vi "StateMachineDAQ.vi"() -> ()   [LabVIEW 2014]
doc: "Use this template to build a user interface event handler design pattern. Use this pattern for dialog boxes and other user interfaces. You also can create and execute user-defined events that the VI can handle the same way as user interface events."
uses:
  subVIs/StateMachineDAQState.ctl
  <vilib>/Utility/error.llb/DialogType.ctl
  <vilib>/DAQmx/create/channels.llb/DAQmx Create Channel (AI-Voltage-Basic).vi
  <vilib>/DAQmx/configure/timing.llb/DAQmx Timing (Sample Clock).vi
  <vilib>/DAQmx/read.llb/DAQmx Read (Analog Wfm 1Chan NSamp).vi
  <resource>/objmgr/daqmx.rc
panel:
  in  "File Path":path
  in  "Acquire Data":bool
  in  "Log Data":bool
  in  "File Comment":string
  in  "DAQ Parameters":T1={"physical channels"="", "maximum value"=5.0, "minimum value"=-5.0, "rate"=1000.0, "read period"=0.5} {"read period" format="%0.2f"; "rate" format="%0.2f"; "minimum value" format="%0.2f"; "maximum value" format="%0.2f"}
  out "Waveform Chart":waveform(dbl)(graph)
  in  "quit":bool
  # "V"
  # "V"
  # "Hz"
  # "s"
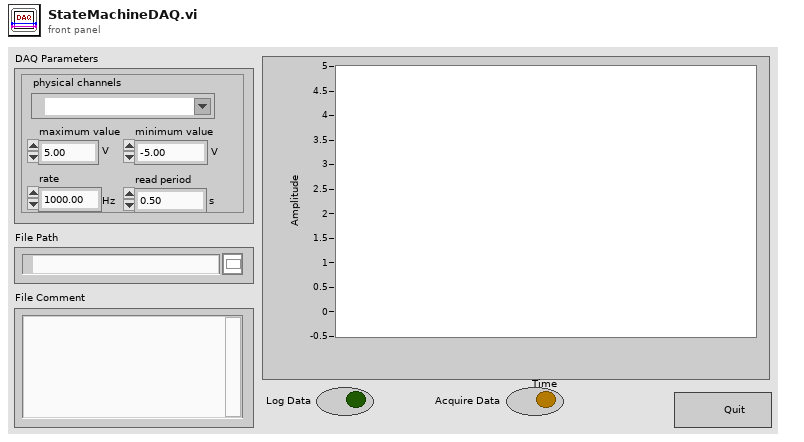
[diagram p1: front panel]
types:
  T1 = cluster{"physical channels":tag, "maximum value":dbl, "minimum value":dbl, "rate":dbl, "read period":dbl}
  T2 = typedef "StateMachineDAQState.ctl" = enum16{"Init", "Idle", "CheckError", "Finalize", "ConfigDAQ", "StartDAQ", "AcquireAndLog", "StopDAQ", "ClearDAQ", "OpenFile", "CloseFile", "Process 1"}
  T3 = typedef "DialogType.ctl" = u16
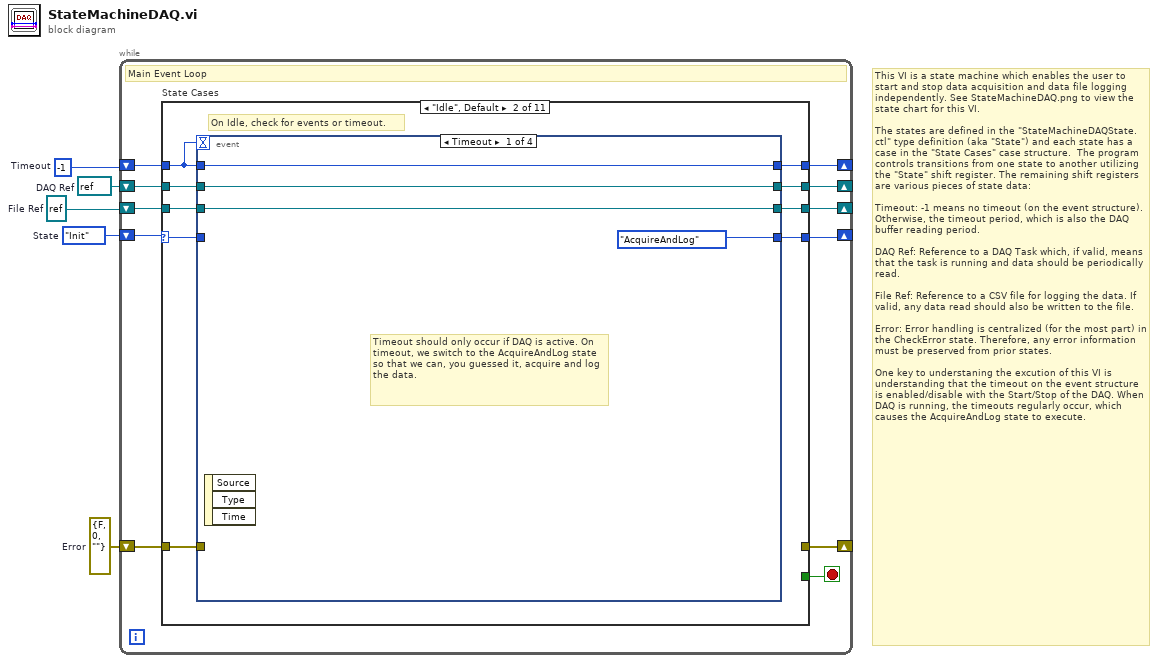
[diagram p0: block diagram]
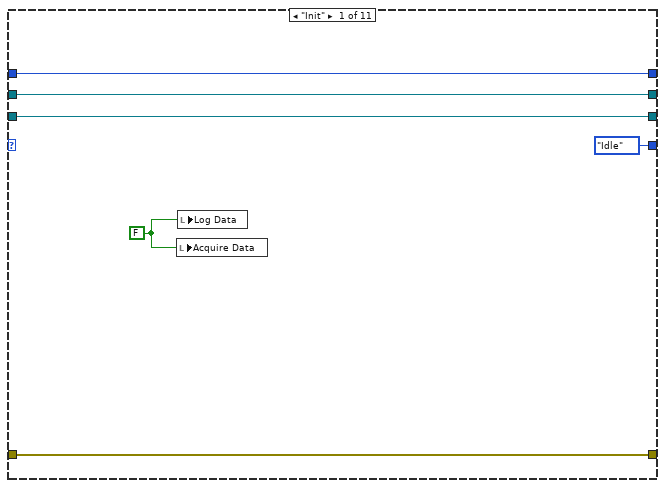
[diagram p2: hidden frame]
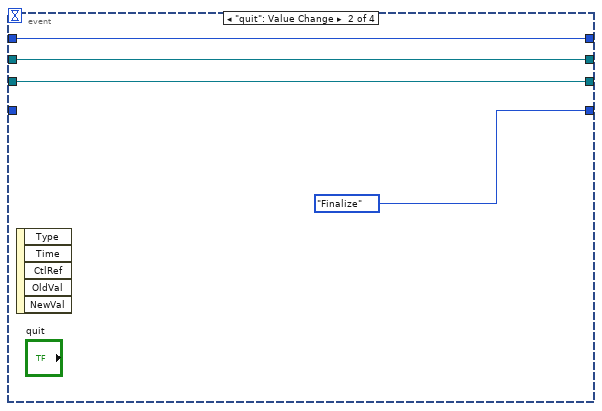
[diagram p3: hidden frame]
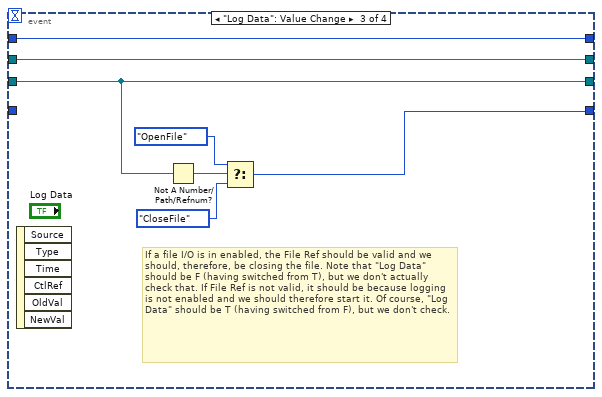
[diagram p4: hidden frame]
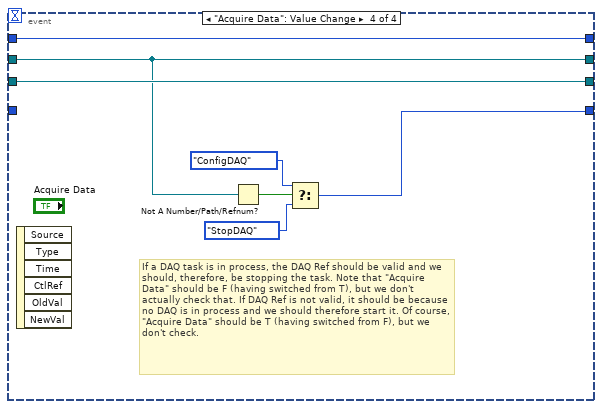
[diagram p5: hidden frame]
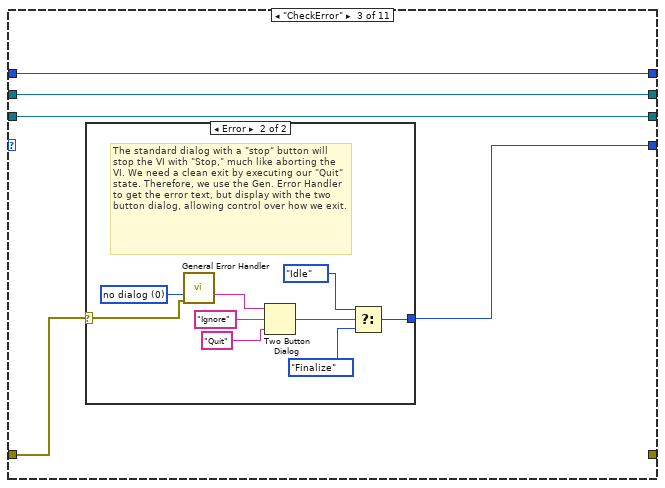
[diagram p6: hidden frame]
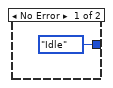
[diagram p7: hidden frame]
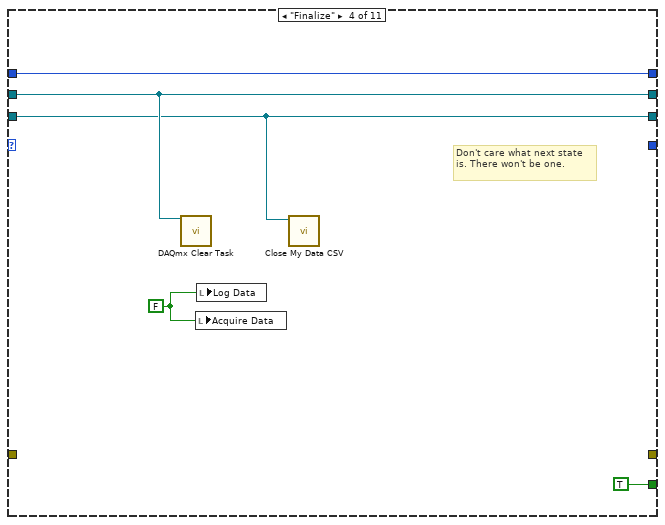
[diagram p8: hidden frame]
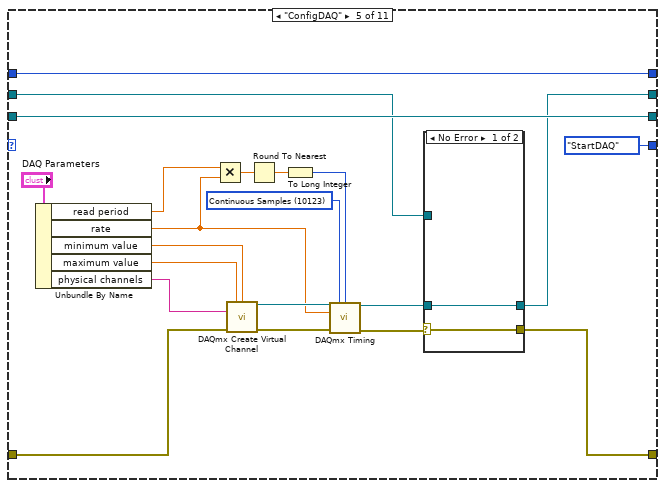
[diagram p9: hidden frame]
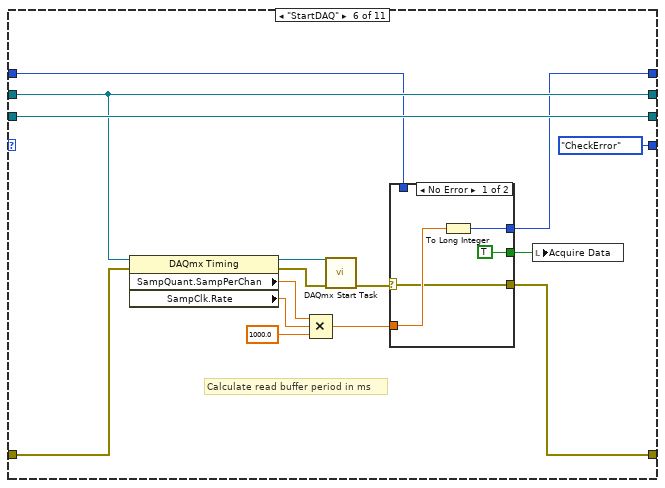
[diagram p11: hidden frame]
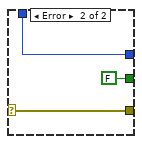
[diagram p12: hidden frame]
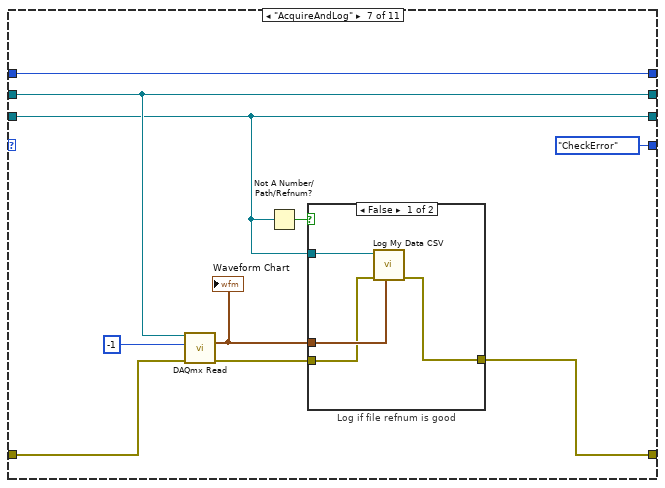
[diagram p13: hidden frame]
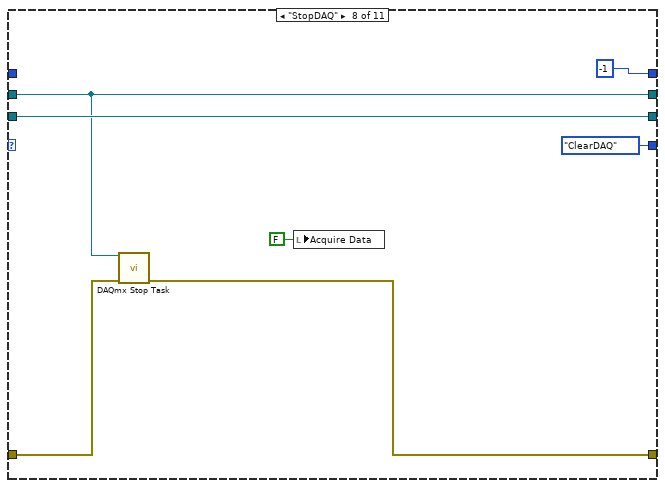
[diagram p15: hidden frame]
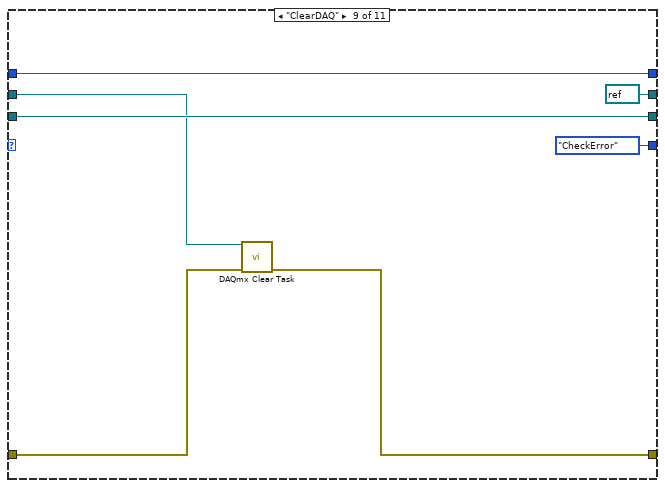
[diagram p16: hidden frame]
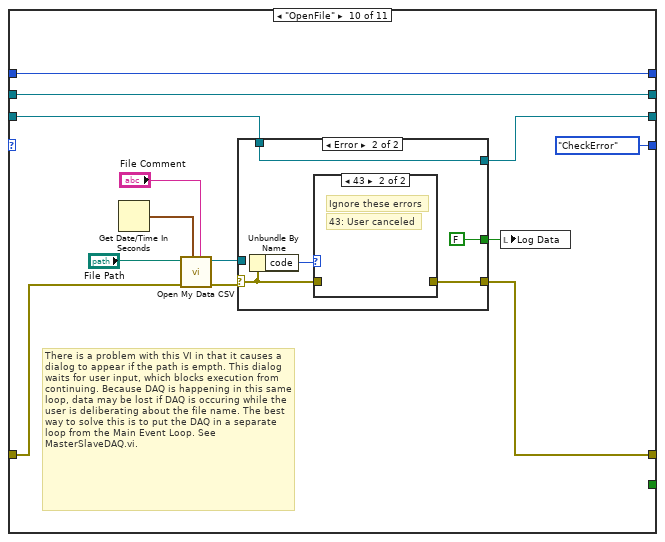
[diagram p17: hidden frame]
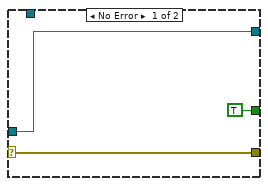
[diagram p18: hidden frame]
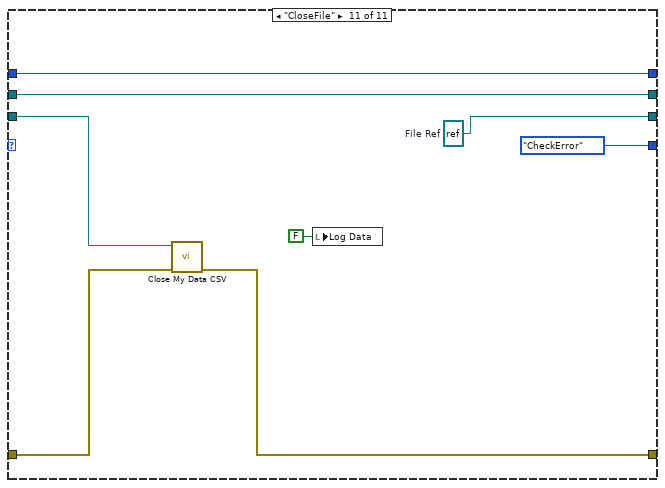
[diagram p20: hidden frame]
diagram:
  w1 = errorcluster {"status"=FALSE, "code"=0, "source"=""}  # Error
  w2 = refnum<file> refnum  # File Ref
  w3 = refnum<k21> refnum  # DAQ Ref
  w4 = StateMachineDAQState."Init"  # State
  w5 = -1  # Timeout
  # "This VI is a state machine which enables the user to start and stop data acquisition and data file logging independently. See StateMachineDAQ.png to view the state chart for this VI.\n\nThe states are defined in the \"StateMachineDAQState.ctl\" type definition (aka \"State\") and each state has a case in the \"State Cases\" case structure.  The program controls transitions from one state to another utilizing the \"State\" shift register. The remaining shift registers are various pieces of state data:\n\nTimeout: -1 means no timeout (on the event structure). Otherwise, the timeout period, which is also the DAQ buffer reading period.\n\nDAQ Ref: Reference to a DAQ Task which, if valid, means that the task is running and data should be periodically read.\n\nFile Ref: Reference to a CSV file for logging the data. If valid, any data read should also be written to the file.\n\nError: Error handling is centralized (for the most part) in the CheckError state. Therefore, any error information must be preserved from prior states.\n\nOne key to understaning the excution of this VI is understanding that the timeout on the event structure is enabled/disable with the Start/Stop of the DAQ. When DAQ is running, the timeouts regularly occur, which causes the AcquireAndLog state to execute."
  n1 = while {
    shift-right: [w15] -> _
    shift-left: w5 -> [w16]
    shift-right: [w13] -> _
    shift-left: w4 -> [w14]
    shift-right: [w12] -> _
    shift-left: w3 -> [w11]
    shift-right: [w10] -> _
    shift-left: w2 -> [w9]
    shift-right: [w8] -> _
    shift-left: w1 -> [w7]
    stop <- w6 stop-if-true
    # "Main Event Loop"
    n2 = case "State Cases" shown="\"Idle\", Default" w14 {
      selector: w14 -> [_ w29 _ _ _ _ _ _ _ _ _]
      tunnel: w16 -> [w22 w31 w58 w73 w82 w108 w126 _ w149 w162 w179]
      tunnel: [w22 w30 w58 w73 w82 w107 w126 -1 ("Timeout") w149 w162 w179] -> w15
      tunnel: [StateMachineDAQState."Idle" ("State") w28 w55 _ StateMachineDAQState."StartDAQ" ("State") StateMachineDAQState."CheckError" ("State") StateMachineDAQState."CheckError" ("State") StateMachineDAQState."ClearDAQ" ("State") StateMachineDAQState."CheckError" ("State") StateMachineDAQState."CheckError" ("State") StateMachineDAQState."CheckError" ("State")] -> w13
      tunnel: [w21 w25 w57 w71 w85 w112 w125 w137 refnum<k21> refnum ("DAQ Ref") w161 w178] -> w12
      tunnel: w11 -> [w21 w24 w57 w71 w86 w112 w125 w137 w145 w161 w178]
      tunnel: [w20 w27 w56 w70 w94 w113 w124 w142 w147 w155 w173] -> w10
      tunnel: w9 -> [w20 w26 w56 w70 w94 w113 w124 w142 w147 w150 w177]
      tunnel: [w17 _ _ _ w83 w106 w123 w138 w143 w154 w175] -> w8
      tunnel: w7 -> [w17 w23 w54 _ w74 w103 w121 w136 w144 w151 w172]
      tunnel: [_ _ _ TRUE _ _ _ _ _ _ _] -> w6
      frame "Init" {
        w18 = FALSE
        n3 = local write "Acquire Data"(w18) -> ()
        n4 = local write "Log Data"(w18) -> ()
      }
      frame "Idle", Default {
        # "On Idle, check for events or timeout."
        # "States"
        n5 = event shown="[0] Timeout" {
          selector: _ -> [_ _ _ _]
          dyn-events: _ -> [_ _ _ _]
          timeout: w31 -> [_ _ _ _]
          tunnel: w31 -> [w35 w39 w46 w53]
          tunnel: [w35 w39 w46 w53] -> w30
          tunnel: w29 -> [_ _ _ _]
          tunnel: [StateMachineDAQState."AcquireAndLog" ("State") StateMachineDAQState."Finalize" ("State") w40 w47] -> w28
          tunnel: [w32 w37 w43 w52] -> w27
          tunnel: w26 -> [w32 w37 w43 w52]
          tunnel: [w34 w38 w45 w50] -> w25
          tunnel: w24 -> [w34 w38 w45 w50]
          tunnel: w23 -> [_ _ _ _]
          event Timeout {
            # "Timeout should only occur if DAQ is active. On timeout, we switch to the AcquireAndLog state so that we can, you guessed it, acquire and log the data."
            n6 = event-data() -> ()  [unwired: 1 in, 3 out]
          }
          event "quit": Value Change {
            n7 = event-data() -> ()  [unwired: 1 in, 5 out]
          }
          event "Log Data": Value Change {
            # "If a file I/O is in enabled, the File Ref should be valid and we should, therefore, be closing the file. Note that \"Log Data\" should be F (having switched from T), but we don't actually check that. If File Ref is not valid, it should be because logging is not enabled and we should therefore start it. Of course, \"Log Data\" should be T (having switched from F), but we don't check."
            n8 = event-data() -> ()  [unwired: 1 in, 6 out]
            n9 = Not A Number/Path/Refnum?(number/path/refnum=w43) -> (NaN/Path/Refnum?=w44:bool)
            n10 = Select(t=StateMachineDAQState."OpenFile" ("State"), s=w44, f=StateMachineDAQState."CloseFile" ("State")) -> (s? t:f=w40:T2)
          }
          event "Acquire Data": Value Change {
            # "If a DAQ task is in process, the DAQ Ref should be valid and we should, therefore, be stopping the task. Note that \"Acquire Data\" should be F (having switched from T), but we don't actually check that. If DAQ Ref is not valid, it should be because no DAQ is in process and we should therefore start it. Of course, \"Acquire Data\" should be T (having switched from F), but we don't check."
            n11 = event-data() -> ()  [unwired: 1 in, 6 out]
            n12 = Not A Number/Path/Refnum?(number/path/refnum=w50) -> (NaN/Path/Refnum?=w51:bool)
            n13 = Select(t=StateMachineDAQState."ConfigDAQ" ("State"), s=w51, f=StateMachineDAQState."StopDAQ" ("State")) -> (s? t:f=w47:T2)
          }
        }
      }
      frame "CheckError" {
        n14 = case shown="Error" w54 {
          selector: w54 -> [_ w60]
          tunnel: [StateMachineDAQState."Idle" ("State") w61] -> w55
          frame No Error {
          }
          frame Error {
            w68 = T3 0 items=["no dialog", "OK message", "continue or stop message", "OK message + warnings", "continue/stop + warnings"] ("type of dialog (OK msg:1)")
            # "The standard dialog with a \"stop\" button will stop the VI with \"Stop,\" much like aborting the VI. We need a clean exit by executing our \"Quit\" state. Therefore, we use the Gen. Error Handler to get the error text, but display with the two button dialog, allowing control over how we exit."
            n15 = call <vilib>:"General Error Handler.vi"("type of dialog (OK msg:1)"=w68, "error in (no error)"=w60) -> ("message"=w67:string)  [unwired: 9 in, 4 out]
            n16 = Two Button Dialog(message=w67, 1:"Quit" ("F button name (\"Cancel\")"), 2:"Ignore" ("T button name (\"OK\")")) -> (T button?=w64:bool)
            n17 = Select(t=StateMachineDAQState."Idle" ("State"), s=w64, f=StateMachineDAQState."Finalize" ("State")) -> (s? t:f=w61:T2)
          }
        }
      }
      frame "Finalize" {
        w69 = FALSE
        # "Don't care what next state is. There won't be one."
        n18 = call <vilib>:"DAQmx Clear Task.vi"("task in"=w71) -> ()  [unwired: 14 in, 1 out]
        n19 = local write "Acquire Data"(w69) -> ()
        n20 = local write "Log Data"(w69) -> ()
        n21 = call "Close My Data CSV.vi"("file refnum"=w70) -> ()  [unwired: 10 in, 1 out]
      }
      frame "ConfigDAQ" {
        w91 = 10123 items=["Finite Samples"=10178, "Continuous Samples"=10123, "Hardware Timed Single Point"=12522] ("sample mode")
        n22 = Unbundle By Name("DAQ Parameters") -> ("read period"=w79:dbl, "rate"=w78:dbl, "minimum value"=w77:dbl, "maximum value"=w76:dbl, "physical channels"=w75:tag)
        n23 = Multiply(x=w79, y=w78) -> (x*y=w90:dbl)
        n24 = call-poly <vilib>:"DAQmx Create Virtual Channel.vi"("maximum value"=w76, "minimum value"=w77, "physical channels"=w75, "error in"=w74) -> ("task out"=w93:refnum<k21>, "error out"=w92:errorcluster)  [unwired: 10 in]
        n25 = Round To Nearest(number=w90) -> (nearest integer value=w89:dbl)
        n26 = To Long Integer(number=w89) -> (32bit integer=w88:i32)
        n27 = call-poly <vilib>:"DAQmx Timing.vi"("task/channels in"=w93, "sample mode"=w91, "samples per channel"=w88, "rate"=w78, "error in"=w92) -> ("task out"=w84:refnum<k21>, "error out"=w87:errorcluster)  [unwired: 9 in]
        n28 = case shown="No Error" w87 {
          selector: w87 -> [w95 w98]
          tunnel: w86 -> [_ w97]
          tunnel: [w96 w97] -> w85
          tunnel: w84 -> [w96 _]
          tunnel: [w95 w98] -> w83
          frame No Error {
          }
          frame Error {
          }
        }
      }
      frame "StartDAQ" {
        # "Calculate read buffer period in ms"
        n29 = property class="DAQmx Timing"(reference=w112, error in=w103) -> (reference out=w111:refnum<k21>, error out=w110:errorcluster, "SampQuant.SampPerChan"=w102:dbl, "SampClk.Rate"=w101:dbl)
        n30 = Compound Arithmetic op=MULTIPLY(w102, w101, 1000.0 ("value")) -> (w99:dbl)
        n31 = call <vilib>:"DAQmx Start Task.vi"("task/channels in"=w111, "error in"=w110) -> ("error out"=w109:errorcluster)  [unwired: 12 in, 1 out]
        n32 = case shown="No Error" w109 {
          selector: w109 -> [w115 w119]
          tunnel: w99 -> [w117 _]
          tunnel: w108 -> [_ w120]
          tunnel: [w116 w120] -> w107
          tunnel: [w115 w119] -> w106
          tunnel: [TRUE FALSE] -> w104
          frame No Error {
            n33 = To Long Integer(number=w117) -> (32bit integer=w116:i32)
          }
          frame Error {
          }
        }
        n34 = local write "Acquire Data"(w104) -> ()
      }
      frame "AcquireAndLog" {
        n35 = call-poly <vilib>:"DAQmx Read.vi"("task/channels in"=w125, "number of samples per channel"=-1, "error in"=w121) -> ("data"=w127:waveform(dbl), "error out"=w128:errorcluster)  [unwired: 10 in, 1 out]
        "Waveform Chart" <- w127
        n36 = Not A Number/Path/Refnum?(number/path/refnum=w124) -> (NaN/Path/Refnum?=w129:bool)
        n37 = case "Log if file refnum is good" shown="False" w129 {
          tunnel: w128 -> [w132 w135]
          tunnel: w124 -> [w134 _]
          tunnel: w127 -> [w133 _]
          tunnel: [w131 w135] -> w123
          frame False {
            n38 = call "Log My Data CSV.vi"("Data"=w133, "error in"=w132, "file refnum"=w134) -> ("error out"=w131:errorcluster)  [unwired: 7 in, 1 out]
          }
          frame True {
          }
        }
      }
      frame "StopDAQ" {
        n39 = call <vilib>:"DAQmx Stop Task.vi"("task/channels in"=w137, "error in"=w136) -> ("error out"=w138:errorcluster)  [unwired: 12 in, 1 out]
        n40 = local write "Acquire Data"(FALSE ("Acquire Data")) -> ()
      }
      frame "ClearDAQ" {
        n41 = call <vilib>:"DAQmx Clear Task.vi"("task in"=w145, "error in"=w144) -> ("error out"=w143:errorcluster)  [unwired: 13 in]
      }
      frame "OpenFile" {
        # "There is a problem with this VI in that it causes a dialog to appear if the path is empth. This dialog waits for user input, which blocks execution from continuing. Because DAQ is happening in this same loop, data may be lost if DAQ is occuring while the user is deliberating about the file name. The best way to solve this is to put the DAQ in a separate loop from the Main Event Loop. See MasterSlaveDAQ.vi."
        n42 = Get Date/Time In Seconds() -> (seconds since 1Jan1904=w160:timestamp)
        n43 = call "Open My Data CSV.vi"("Comment"="File Comment", "Time Stamp"=w160, "error in"=w151, "file path"="File Path") -> ("error out"=w157:errorcluster, "refnum out"=w156:refnum<file>)  [unwired: 6 in]
        n44 = case shown="Error" w157 {
          selector: w157 -> [w164 w167]
          tunnel: [w165 w169] -> w155
          tunnel: w156 -> [w165 _]
          tunnel: [w164 w166] -> w154
          tunnel: [TRUE ("Log Data") FALSE ("Log Data")] -> w153
          tunnel: w150 -> [_ w169]
          frame No Error {
          }
          frame Error {
            n45 = Unbundle By Name(w167) -> ("code"=w168:i32)
            n46 = case shown="43" w168 {
              tunnel: w167 -> [w171 _]
              tunnel: [w171 _] -> w166
              frame 1, Default {
                # "Process these errors"
              }
              frame 43 {
                # "43: User canceled"
                # "Ignore these errors"
              }
            }
          }
        }
        n47 = local write "Log Data"(w153) -> ()
      }
      frame "CloseFile" {
        w173 = refnum<file> refnum  # File Ref
        n48 = call "Close My Data CSV.vi"("error in"=w172, "file refnum"=w177) -> ("error out"=w175:errorcluster)  [unwired: 9 in]
        n49 = local write "Log Data"(FALSE ("Log Data")) -> ()
      }
    }
  }
